vi "Adjust Mark10 Speed.vi"(8 "error in (no error)":errorcluster, 10 "load test?":bool, 11 "Requested Speed":dbl) -> (0 "error out":errorcluster, 3 "Cmds":string[](array[string]))   [LabVIEW 2015]
uses:
  Controls/Mark10 Comm states.ctl
panel:
  in  "SpeedLimit":cluster{"Max":dbl, "Min":dbl}={"Max"=32.0, "Min"=0.0}
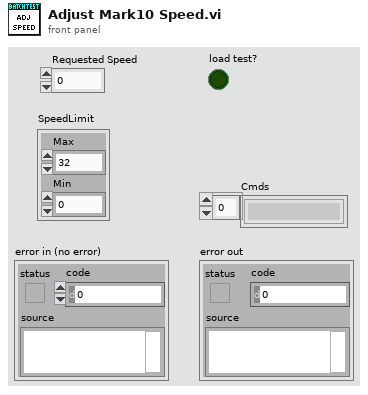
[diagram p1: front panel]
types:
  T1 = typedef "Mark10 Comm states.ctl" = enum16{"Open Session", "Get Reference", "Write Data", "Read Data", "Close Session"}
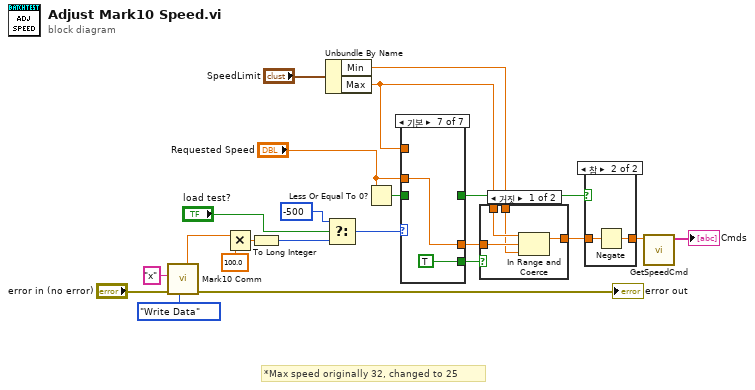
[diagram p0: block diagram]
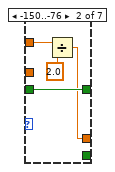
[diagram p5: hidden frame]
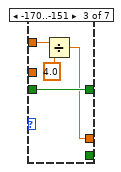
[diagram p6: hidden frame]
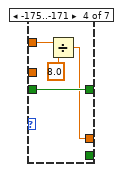
[diagram p7: hidden frame]
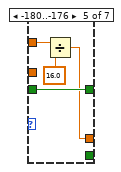
[diagram p8: hidden frame]
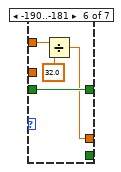
[diagram p9: hidden frame]
diagram:
  # "*Max speed originally 32, changed to 25"
  n1 = call "Mark10 Comm.vi"("Action"=Mark10_Comm_states."Write Data", "error in (no error)"="error in (no error)", "Write"="x") -> ("error out"=→"error out":errorcluster, "Position"=w18:dbl)  [unwired: 2 in, 5 out]
  n2 = Multiply(x=w18, y=100.0) -> (x*y=w16:dbl)
  n3 = To Long Integer(number=w16) -> (32bit integer=w3:i32)
  n4 = Unbundle By Name("SpeedLimit") -> ("Min"=w5:dbl, "Max"=w6:dbl)
  n5 = Select(t=-500, s="load test?", f=w3) -> (s? t:f=w2:i32)
  n6 = Less Or Equal To 0?(x="Requested Speed") -> (x <= 0?=w21:bool)
  n7 = case shown="기본" w2 {
    tunnel: [w23 w25 w29 w33 w37 w41 w46] -> w10
    tunnel: "Requested Speed" -> [_ _ _ _ _ _ w46]
    tunnel: w21 -> [w24 w28 w32 w36 w40 w44 _]
    tunnel: [w24 w28 w32 w36 w40 w44 _] -> w22
    tunnel: [_ _ _ _ _ _ TRUE] -> w8
    tunnel: w6 -> [w23 w27 w30 w34 w38 w42 _]
    frame -75.. {
    }
    frame -150..-76 {
      n8 = Divide(x=w27, y=2.0) -> (x/y=w25:dbl)
    }
    frame -170..-151 {
      n9 = Divide(x=w30, y=4.0) -> (x/y=w29:dbl)
    }
    frame -175..-171 {
      n10 = Divide(x=w34, y=8.0) -> (x/y=w33:dbl)
    }
    frame -180..-176 {
      n11 = Divide(x=w38, y=16.0) -> (x/y=w37:dbl)
    }
    frame -190..-181 {
      n12 = Divide(x=w42, y=32.0) -> (x/y=w41:dbl)
    }
    frame Default {
    }
  }
  n13 = case shown="거짓" w8 {
    tunnel: w10 -> [w50 w51]
    tunnel: [w49 w51] -> w9
    tunnel: w6 -> [w48 _]
    tunnel: w5 -> [w47 _]
    frame False {
      n14 = In Range and Coerce(upper limit=w48, x=w50, lower limit=w47) -> (coerced(x)=w49:dbl)  [unwired: 1 out]
    }
    frame True {
    }
  }
  n15 = case shown="참" w22 {
    tunnel: w9 -> [w52 w54]
    tunnel: [w52 w53] -> w20
    frame False {
    }
    frame True {
      n16 = Negate(x=w54) -> (-x=w53:dbl)
    }
  }
  n17 = call "GetSpeedCmd.vi"("Speed"=w20) -> ("Cmds"=→"Cmds":string[])  [unwired: 10 in]
